vi "_Test_RDBAPI.vi"() -> ()   [LabVIEW 2023]
uses:
  RDB/RDB Object.ctl
  RDB/RDB Player Object.ctl
  RDB/RDB Reference.ctl
  <vilib>/xnet/xnet.llb/XNET Frame FlexRay.ctl
  <vilib>/xnet/xnet.llb/XNET Frame Type FlexRay.ctl
  <vilib>/Utility/xml.llb/Read From XML File(string).vi
  RDB/RDB.lvlib
panel:
  out "size(s) 2":i32
  out "size(s)":i32
  out "Array 2":u8[](array[numeric])
  out "Array":i32[](array[numeric])
  out "signal data":dbl[](array[numeric])
  out "simTime":dbl
  out "simFrame":dbl
  out "RDB Reference":T1 {"RDB Data"."payload" format="%x"; "RDB Data"."timestamp" format="%<%.7X\n%x>T"; "RDB Data"."type" items=["FlexRay Data"=32, "FlexRay Null"=33, "FlexRay Symbol"=34, "Log Trigger"=225, "Start Trigger"=226]; "RDB Data"."cycle count" max=63 step=1}
  out "value":T4[](array[typedef])
  in  "XML File Path":path=path "C:/Debug/Receive.xml"
  out "error out":errorcluster
  in  "error in (no error)":errorcluster
  in  "path in":path=path "C:/dev/Hexagon-VTD-Custom-Device/Libraries/libVC.dll"
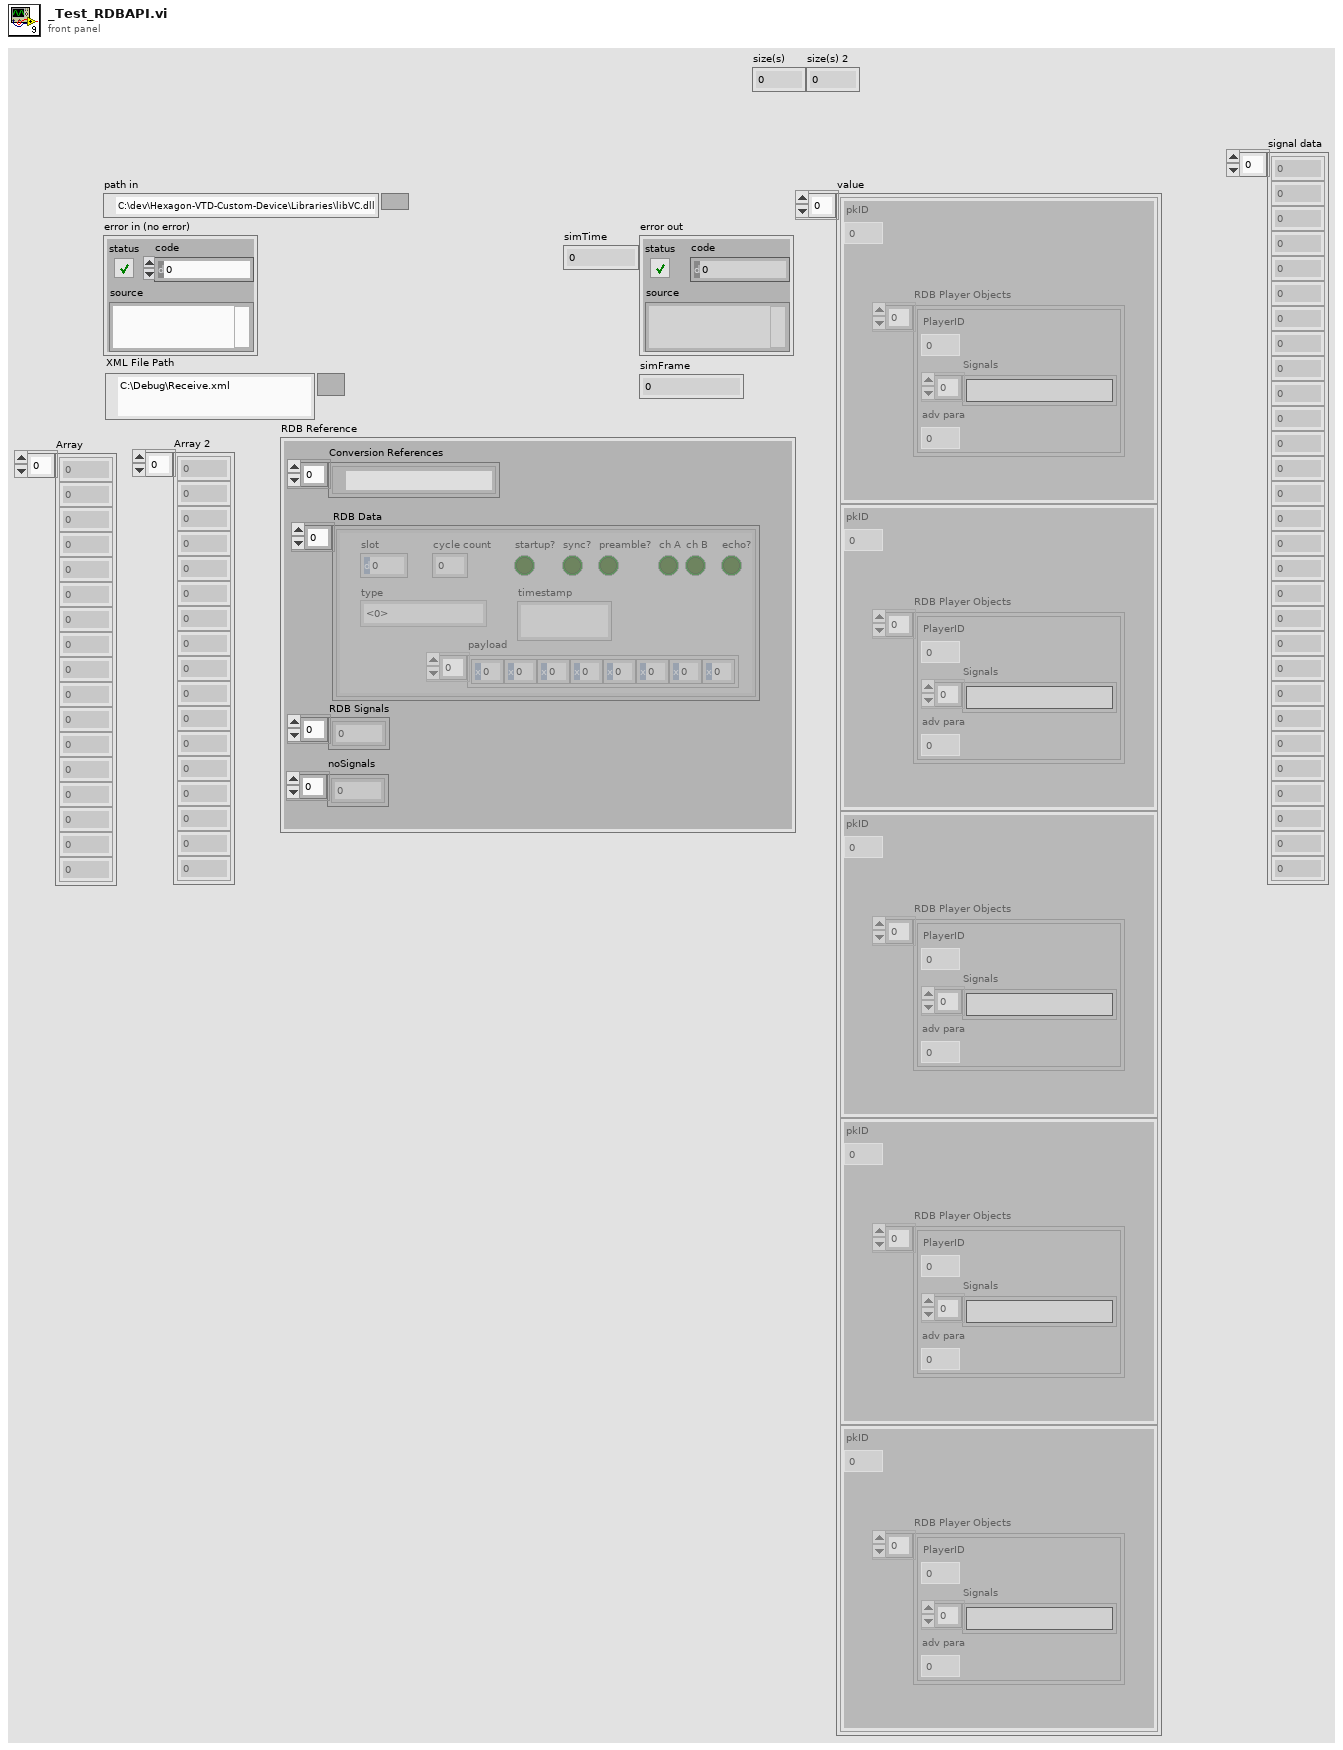
[diagram p1: front panel]
types:
  T1 = typedef "RDB.lvlib/RDB Reference.ctl" = cluster{"Conversion References":refnum<k21>[], "RDB Data":T2[], "RDB Signals":dbl[], "noSignals":i32[]}
  T2 = typedef "XNET Frame FlexRay.ctl" = cluster{"timestamp":timestamp, "payload":u8[], "slot":u16, "type":T3, "cycle count":u8, "startup?":bool, "sync?":bool, "preamble?":bool, "ch A":bool, "ch B":bool, "echo?":bool}
  T3 = typedef "XNET Frame Type FlexRay.ctl" = u8
  T4 = typedef "RDB.lvlib/RDB Object.ctl" = cluster{"pkID":i32, "RDB Player Objects":T5[]}
  T5 = typedef "RDB.lvlib/RDB Player Object.ctl" = cluster{"PlayerID":i32, "Signals":string[], "adv para":i32}
  T6 = enum16{"Standard", "Buffered", "CRLF", "Immediate"}
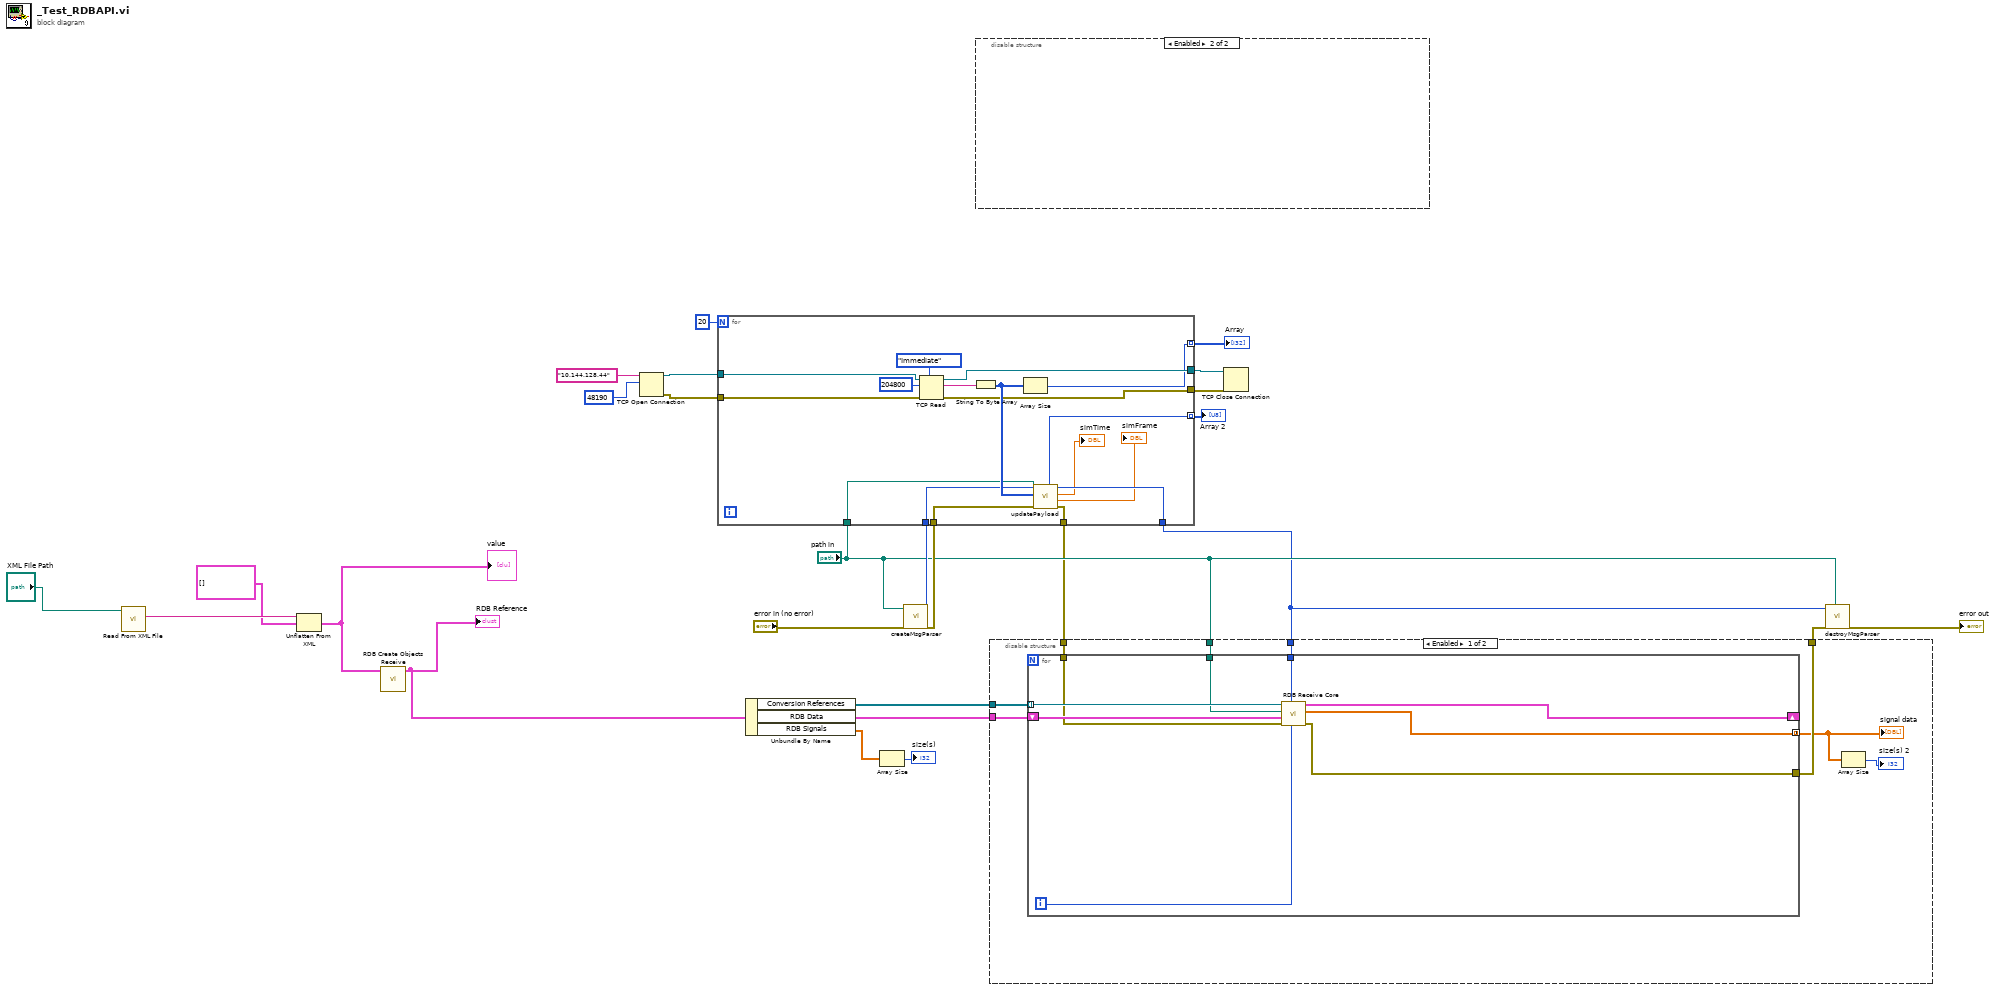
[diagram p0: block diagram]
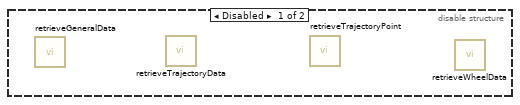
[diagram p3: hidden frame]
diagram:
  n1 = call-poly <vilib>:"Read From XML File.vi"("XML File Path"="XML File Path") -> ("XML Elements"=w24:string)  [unwired: 8 in, 2 out]
  n2 = Unflatten From XML(xml string=w24, type=T4[] []) -> (value=w21:T4[])  [unwired: 1 in, 1 out]
  "value" <- w21
  n3 = call "RDB Create Objects Receive.vi"("RDB Data Receive"=w21) -> ("RDB Reference"=w20:T1)  [unwired: 9 in, 1 out]
  "RDB Reference" <- w20
  n4 = TCP Open Connection(address="10.144.128.44", remote port or service name=u16 48190) -> (connection ID=w14:refnum<k5>, error out=w15:errorcluster)  [unwired: 3 in]
  n5 = Unbundle By Name(w20) -> ("Conversion References"=w11:refnum<k21>[], "RDB Data"=w10:T2[], "RDB Signals"=w2:dbl[])
  n6 = Array Size(array=w2) -> (size(s)=→"size(s)":i32)
  n7 = call "createMsgParser.vi"("error in (no error)"="error in (no error)", "path in"="path in") -> ("error out"=w19:errorcluster, "paeseHandle"=w18:u64)  [unwired: 8 in]
  n8 = for {
    N: 20 -> [_]
    tunnel: "path in" -> [w39]
    tunnel: w19 -> [w38]
    tunnel: w18 -> [w37]
    tunnel: [w36] -> w8
    tunnel: [w35] -> w5
    tunnel: w15 -> [w34]
    tunnel: w14 -> [w33]
    tunnel: [w32] -> w13
    tunnel: [w31] -> w12
    tunnel: [w28] -> w4 mode=indexing
    tunnel: [w27] -> w3 mode=indexing
    n9 = TCP Read(connection ID=w33, bytes to read=204800, error in (no error)=w34, 7:T6."Immediate" ("mode (standard)")) -> (connection ID out=w32:refnum<k5>, data out=w42:string, error out=w31:errorcluster)  [unwired: 1 in]
    n10 = String To Byte Array(string=w42) -> (unsigned byte array=w40:u8[])
    n11 = Array Size(array=w40) -> (size(s)=w28:i32)
    n12 = call "updatePayload.vi"("path in"=w39, "error in (no error)"=w38, "payload"=w40, "paeseHandle in"=w37) -> ("error out"=w36:errorcluster, "simFrame"=→"simFrame":dbl, "simTime"=→"simTime":dbl, "paeseHandle out"=w35:u64, "isComplete"=w27:u8)  [unwired: 3 in]
  }
  "Array" <- w4
  "Array 2" <- w3
  n13 = disable-structure shown="Enabled" {
    frame Disabled {
      n14 = call "retrieveGeneralData.vi"() -> ()  [unwired: 13 in, 3 out]
      n15 = call "retrieveTrajectoryData.vi"() -> ()  [unwired: 13 in, 3 out]
      n16 = call "retrieveTrajectoryPoint.vi"() -> ()  [unwired: 13 in, 3 out]
      n17 = call "retrieveWheelData.vi"() -> ()  [unwired: 13 in, 3 out]
    }
    frame Enabled {
    }
  }
  n18 = disable-structure shown="Enabled" {
    disable-tunnel: w11 -> [w51 _]
    disable-tunnel: w10 -> [w50 _]
    disable-tunnel: "path in" -> [w49 _]
    disable-tunnel: w8 -> [w48 w61]
    disable-tunnel: [w47 w61] -> w7
    disable-tunnel: w5 -> [w46 _]
    frame Enabled {
      n19 = for {
        tunnel: w51 -> [w59] mode=indexing
        tunnel: [w56] -> w45 mode=concatenating
        shift-right: [w57] -> _
        shift-left: w50 -> [w58]
        tunnel: w49 -> [w55]
        tunnel: w48 -> [w54]
        tunnel: [w53] -> w47
        tunnel: w46 -> [w52]
        i -> [w60]
        n20 = call "RDB Receive Core.vi"("index"=w60, "paeseHandle in"=w52, "error in (no error)"=w54, "RDB Data in"=w58, "vclient"=w55, "XNET Conversion"=w59) -> ("error out"=w53:errorcluster, "signal data"=w56:dbl[], "RDB Data out"=w57:T2[])  [unwired: 3 in]
      }
      "signal data" <- w45
      n21 = Array Size(array=w45) -> (size(s)=→"size(s) 2":i32)
    }
    frame Disabled {
    }
  }
  n22 = TCP Close Connection(connection ID=w13, error in (no error)=w12) -> ()  [unwired: 1 in, 2 out]
  n23 = call "destroyMsgParser.vi"("path in"="path in", "error in (no error)"=w7, "parserHandle"=w5) -> ("error out"=→"error out":errorcluster)  [unwired: 8 in]
